vi "GenerateTestImageCPUTrack.vi"(0 "width":u32=256, 1 "height":u32=256, 2 "image":T1, 3 "xpos":sgl=128.0, 4 "ypos":sgl=128.0, 6 "spotsize":sgl=20.0) -> (5 "Image":T1(plugin-control))   [LabVIEW 2011]
uses:
  <vilib>/vision/Image Controls.llb/IMAQ Image.ctl
  CpuTrackDLL.vi
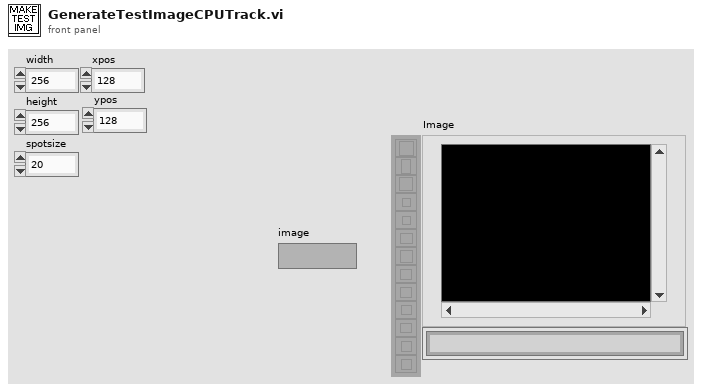
[diagram p1: front panel]
types:
  T1 = typedef "IMAQ Image.ctl" = refnum<image>
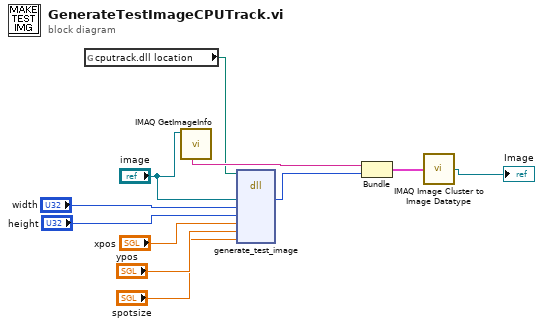
[diagram p0: block diagram]
diagram:
  n1 = global read "CpuTrackDLL.vi" "cputrack.dll location"() -> (w1:path)
  n2 = call "IMAQ GetImageInfo"("Image"="image") -> ("Image Name"=w5:string)  [unwired: 3 in, 7 out]
  n3 = dll-call lib="D:/jcnossen1/cudaqi-tracker/cputrack/cputrack_d.dll" fn="generate_test_image"(path in=w1, "image"="image", "width"="width", "height"="height", "xpos"="xpos", "ypos"="ypos", "spotsize"="spotsize") -> ("image"=w3:u64)  [unwired: 8 in, 2 out]
  n4 = Bundle("Image Name"=w5, "image"=w3) -> (w6:cluster{"Image Name":string, "image":u64})  [unwired: 1 in]
  n5 = call <vilib>:"IMAQ Image Cluster to Image Datatype.vi"("Image"=w6) -> ("Image (dup)"=→"Image":T1)
